vi "Resample Waveform (single shot, t0 DBL).vi"(0 "waveform in":waveform(dbl), 1 "open interval? (T)":bool=TRUE, 5 "dt":dbl=1.0 format="%.2p", 7 "t0":dbl=-inf format="%.2p", 9 "interpolation mode":u16(ring)=1 items=["coerce", "linear", "spline", "FIR filter"], 11 "error in (no error)":errorcluster, 12 "FIR filter specifications":T1={"alias rejection (dB)"=120.0, "normalized bandwidth"=0.4536} {"normalized bandwidth" format="%.4f"; "alias rejection (dB)" format="%.2f"}) -> (4 "resampled waveform out":waveform(dbl), 10 "used t0":dbl format="%.2p", 14 "t0 adjusted warning":bool, 15 "error out":errorcluster)   [LabVIEW 2020, in "NI_MAPro.lvlib"]
doc: "Resamples input waveforms or data according to the user-defined <B>t0</B> and <B>dt</B> values. You can use this polymorphic VI to resample a single waveform, N waveforms, an array of XY pairs, a pair of X and Y arrays, N arrays of XY pairs, or N pairs of X and Y arrays. The data type you wire to the waveform or data input determines the polymorphic instance to use."
uses:
  NI_MAPro.lvlib
panel:
  # "open"
  # "closed"
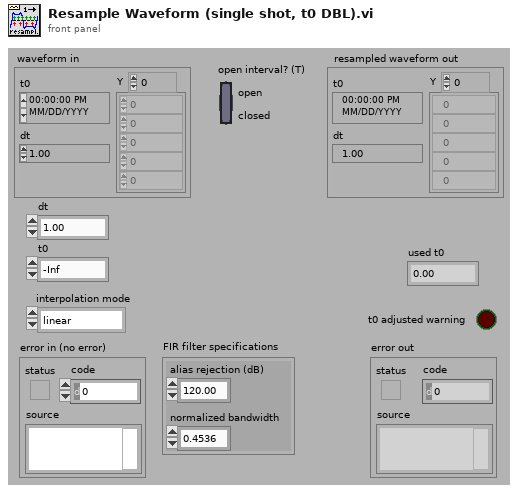
[diagram p1: front panel]
types:
  T1 = cluster{"alias rejection (dB)":dbl, "normalized bandwidth":dbl}
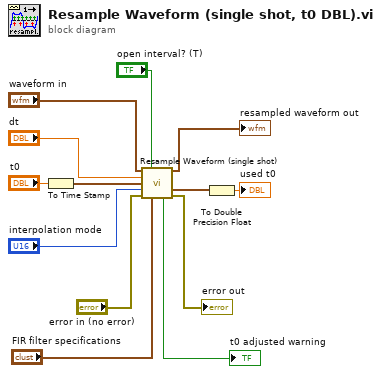
[diagram p0: block diagram]
diagram:
  n1 = To Time Stamp(1:"t0") -> (0:w5:timestamp)
  n2 = call "Resample Waveform (single shot).vi"("waveform in"="waveform in", "open interval? (F)"="open interval? (T)", "dt"="dt", "t0"=w5, "interpolation mode"="interpolation mode", "error in (no error)"="error in (no error)", "FIR filter specifications"="FIR filter specifications") -> ("resampled waveform out"=→"resampled waveform out":waveform(dbl), "used t0"=w2:timestamp, "t0 adjusted warning"=→"t0 adjusted warning":bool, "error out"=→"error out":errorcluster)  [unwired: 5 in]
  n3 = To Double Precision Float(number=w2) -> (double precision float=→"used t0":dbl)
